vi "SCAN.vi"(0 "refnum in":refnum<vi>, 1 "Cursor":string, 5 "Use Pattern ?":bool, 7 "Pattern":string, 11 "error in":errorcluster, 12 "Use Count ?":bool, 13 "Count":string) -> (4 "refnum out":refnum<vi>, 6 "Data":T1, 15 "error out":errorcluster)   [LabVIEW 2020]
uses:
  SubVIs/Controls/redis-data.ctl
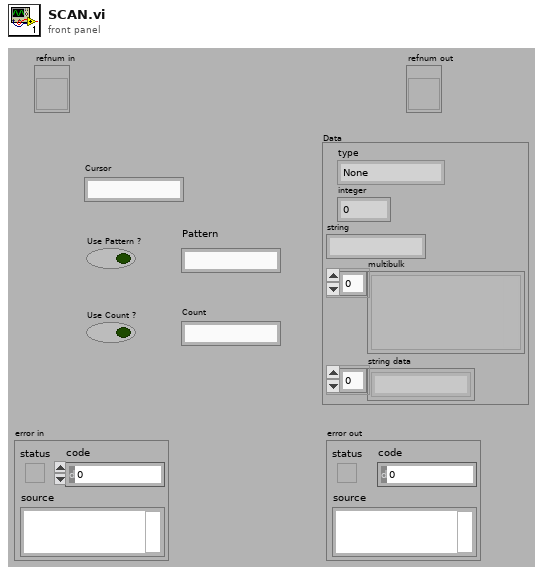
[diagram p1: front panel]
types:
  T1 = typedef "redis-data.ctl" = cluster{"type":enum16{"None", "Error", "Status", "Nil", "Integer", "String", "Multibulk"}, "integer":i64, "string":string, "multibulk":variant[], "string data":string[]}
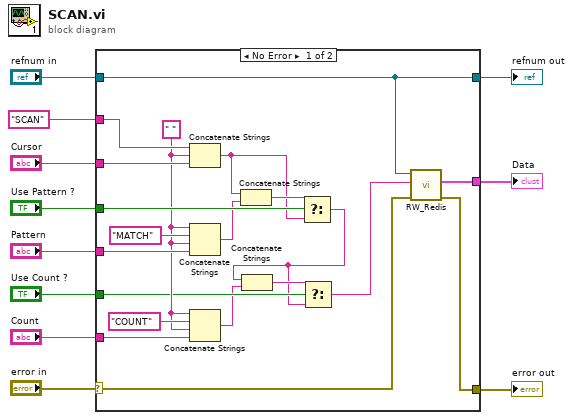
[diagram p0: block diagram]
diagram:
  n1 = case shown="No Error" "error in" {
    selector: "error in" -> [w30 w33]
    tunnel: "Cursor" -> [w27 _]
    tunnel: "SCAN" -> [w31 _]
    tunnel: "refnum in" -> [w12 w32]
    tunnel: [w29 w33] -> w9
    tunnel: [w28 _] -> w1
    tunnel: "Pattern" -> [w26 _]
    tunnel: "Use Pattern ?" -> [w24 _]
    tunnel: "Use Count ?" -> [w16 _]
    tunnel: "Count" -> [w21 _]
    tunnel: [w12 w32] -> w3
    frame No Error {
      w22 = " "
      n2 = Concatenate Strings(w31, w22, w27) -> (w19:string)
      n3 = Concatenate Strings(w22, "MATCH", w22, w26) -> (w18:string)
      n4 = Concatenate Strings(w22, "COUNT", w22, w21) -> (w14:string)
      n5 = Concatenate Strings(w19, w18) -> (w20:string)
      n6 = Select(t=w20, s=w24, f=w19) -> (s? t:f=w15:string)
      n7 = Concatenate Strings(w15, w14) -> (w17:string)
      n8 = Select(t=w17, s=w16, f=w15) -> (s? t:f=w13:string)
      n9 = call "RW_Redis.vi"("error in"=w30, "command"=w13, "refnum"=w12) -> ("error out"=w29:errorcluster, "Data"=w28:T1)  [unwired: 7 in]
    }
    frame Error {
    }
  }
  "error out" <- w9
  "Data" <- w1
  "refnum out" <- w3
